vi "Main1.vi"() -> ()   [LabVIEW 2017]
uses:
  <vilib>/Analysis/baseanly.llb/Mean (DBL).vi
  <vilib>/Analysis/NI_AALBase.lvlib
panel:
  out "file path":path=path "M:/Oceanoptics/TDMS test/Spectrometer_test213.tdms"
  out "Image Out":T1(plugin-control)
  out "String":string
  in  "Save Raw Spectrometer Data":bool=TRUE
  out "Spectrometer Data":T2={[750.0, 800.0], "mean"=-22.554463094146342, array[2540 elements], array[2540 elements], "Color Temperatures"=[[-3182.0998200450113], [-4677.963743364752], [-7826.4943596651665]]}
  out "Voltage Average":dbl
  in  "Wait time (ms)":i32=250
  out "Motor Cluster":cluster{"Motor Relative":dbl[]}={"Motor Relative"=[0.0900112499774972, 0.0, 0.0, 0.0]}
  in  "WL2":dbl=800.0 format="%#_13g"
  in  "WL1":dbl=750.0 format="%#_13g"
  in  "Y axis":T3(ring)=enum."Spectrometer intensity"
  in  "Clear data":bool
  in  "Vi Selection":bool[](array[boolean])=[FALSE, TRUE, TRUE, TRUE, FALSE, TRUE]
  in  "base path":path=path "E:/Materials Testing"
  in  "stop":bool
  out "XY Graph":cluster{"magnitude":dbl[], dbl[]}(graph)
  in  "X axis":T4(ring)=enum."Spectrometer Wavelength"
  # "Power Meter"
  # "Spectrometer"
  # "Sensors"
  # "Motor"
  # "Keithley"
  # "Imaging"
  # "Fluke"
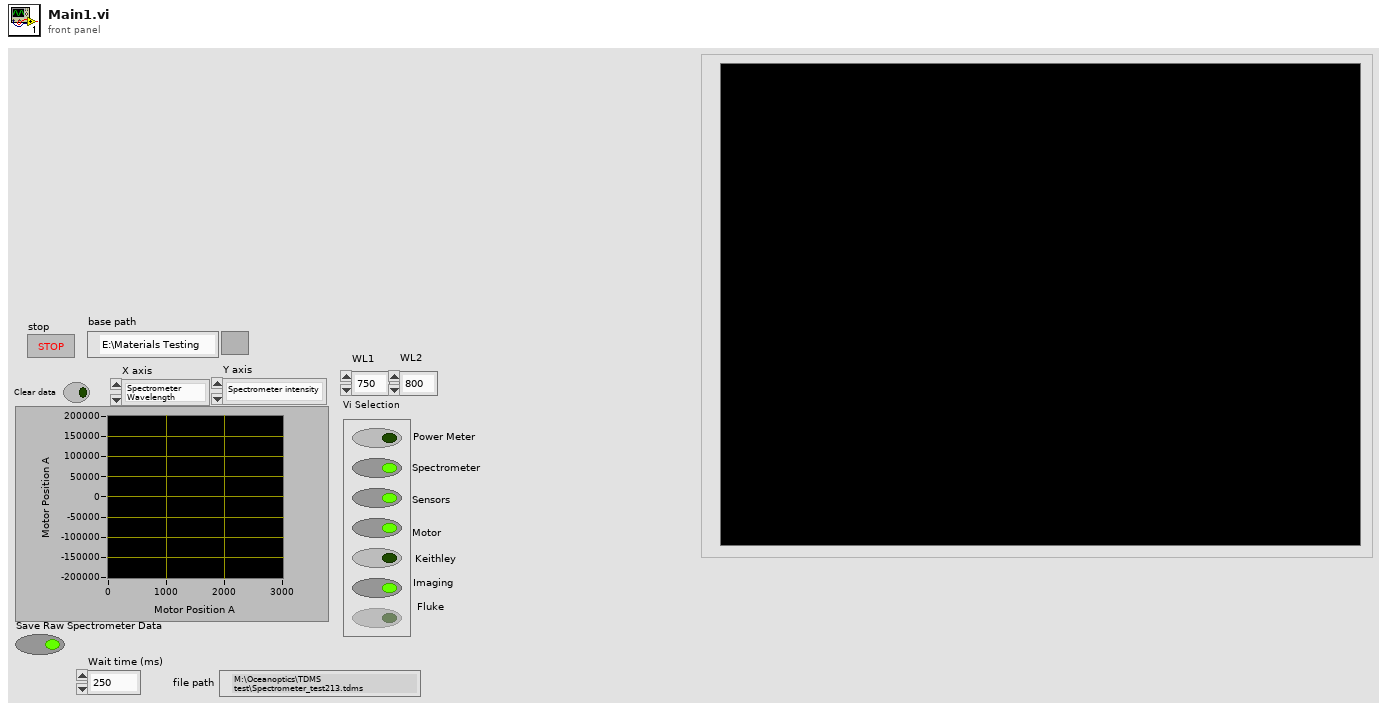
[diagram p1: front panel]
types:
  T1 = typedef "IMAQ Image.ctl" = refnum<image>
  T2 = cluster{dbl[], "mean":dbl, dbl[], dbl[], "Color Temperatures":dbl[][]}
  T3 = enum16{"Motor Position A", "Motor Position B", "Motor Position C", "Motor Position D", "Spectrometer Region Avg.", "Keithley Voltage", "Spectrometer intensity", "Color Temp 2 -3", "Color Temp 1-3", "Color Temp 1-2"}
  T4 = enum16{"Time", "Motor Position A", "Motor Position B", "Motor Position C", "Motor Position D", "Spectrometer Wavelength"}
  T5 = enum16{"PowerMeter", "Spectrometer", "Sensors", "Motor", "Keithley", "Imaging", "Fluke"}
  T6 = enum32{"Invalid", "Standard", "Closed", "Hidden", "Minimized", "Maximized"}
  T7 = cluster{"output cluster 2":cluster{"Value:":dbl[], timestamp[], string[][]}, "output cluster 3":cluster{"Value:":dbl[], timestamp[], string[][]}}
  T8 = cluster{"Temperature Data":cluster{"Bandwidth":i32[], "Bandwidth labels":string[], "Color Temperatures":dbl[][], "Wavelength labels":string[], "seconds since 1Jan1904":timestamp}, "Vis Data":cluster{cluster{"visible wl array":dbl[], dbl[]}, cluster{"Vis or NIR":string, "Multiplexer Response":string, "Wavelength Difference Vis (nm)":dbl, "Vis Integration Time (ms)":u32, "Normalization path":path, "Vis background wave":cluster{dbl[], dbl[]}}}, "NIR Data":cluster{cluster{"NIR wl array":dbl[], dbl[]}, cluster{"Vis or NIR":string, "Multiplexer Response":string, "NIR Integration Time (ms)":u32, "Wavelength Difference NIR (nm) ":dbl, "Normalization path":path, "NIR background wave":cluster{dbl[], dbl[]}}}}
  T9 = cluster{dynamicdata, dynamicdata, dynamicdata, "Dynamic Data Type":dynamicdata}
  T10 = cluster{"Motor Relative":dbl[], "Motor absolute":dbl[], "Motor zero":dbl[], "Time between steps":dbl, "Conversion (steps/mm)":dbl[], "Distance  (mm)":dbl[], "run number":i32, "Number of steps":i32}
  T11 = cluster{"mean":dbl, "seconds since 1Jan1904":timestamp}
  T12 = enum32{"Bad", "Idle", "Run top level", "Running"}
  T13 = cluster{"VI out":refnum<vi>, "error out":errorcluster, refnum<vi>, enum16{"PowerMeter", "Spectrometer", "Sensors", "Motor", "Keithley", "Imaging", "Fluke"}, "Run Power meter":bool}
  T14 = cluster{"Bandwidth":i32[], "Bandwidth labels":string[], "Color Temperatures":dbl[][], "Wavelength labels":string[], "seconds since 1Jan1904":timestamp}
  T15 = cluster{cluster{"visible wl array":dbl[], dbl[]}, cluster{"Vis or NIR":string, "Multiplexer Response":string, "Wavelength Difference Vis (nm)":dbl, "Vis Integration Time (ms)":u32, "Normalization path":path, "Vis background wave":cluster{dbl[], dbl[]}}}
  T16 = cluster{cluster{"NIR wl array":dbl[], dbl[]}, cluster{"Vis or NIR":string, "Multiplexer Response":string, "NIR Integration Time (ms)":u32, "Wavelength Difference NIR (nm) ":dbl, "Normalization path":path, "NIR background wave":cluster{dbl[], dbl[]}}}
  T17 = cluster{"Vis or NIR":string, "Multiplexer Response":string, "NIR Integration Time (ms)":u32, "Wavelength Difference NIR (nm) ":dbl, "Normalization path":path, "NIR background wave":cluster{dbl[], dbl[]}}
  T18 = cluster{"Vis or NIR":string, "Multiplexer Response":string, "Wavelength Difference Vis (nm)":dbl, "Vis Integration Time (ms)":u32, "Normalization path":path, "Vis background wave":cluster{dbl[], dbl[]}}
  T19 = typedef "Image Type" = u32
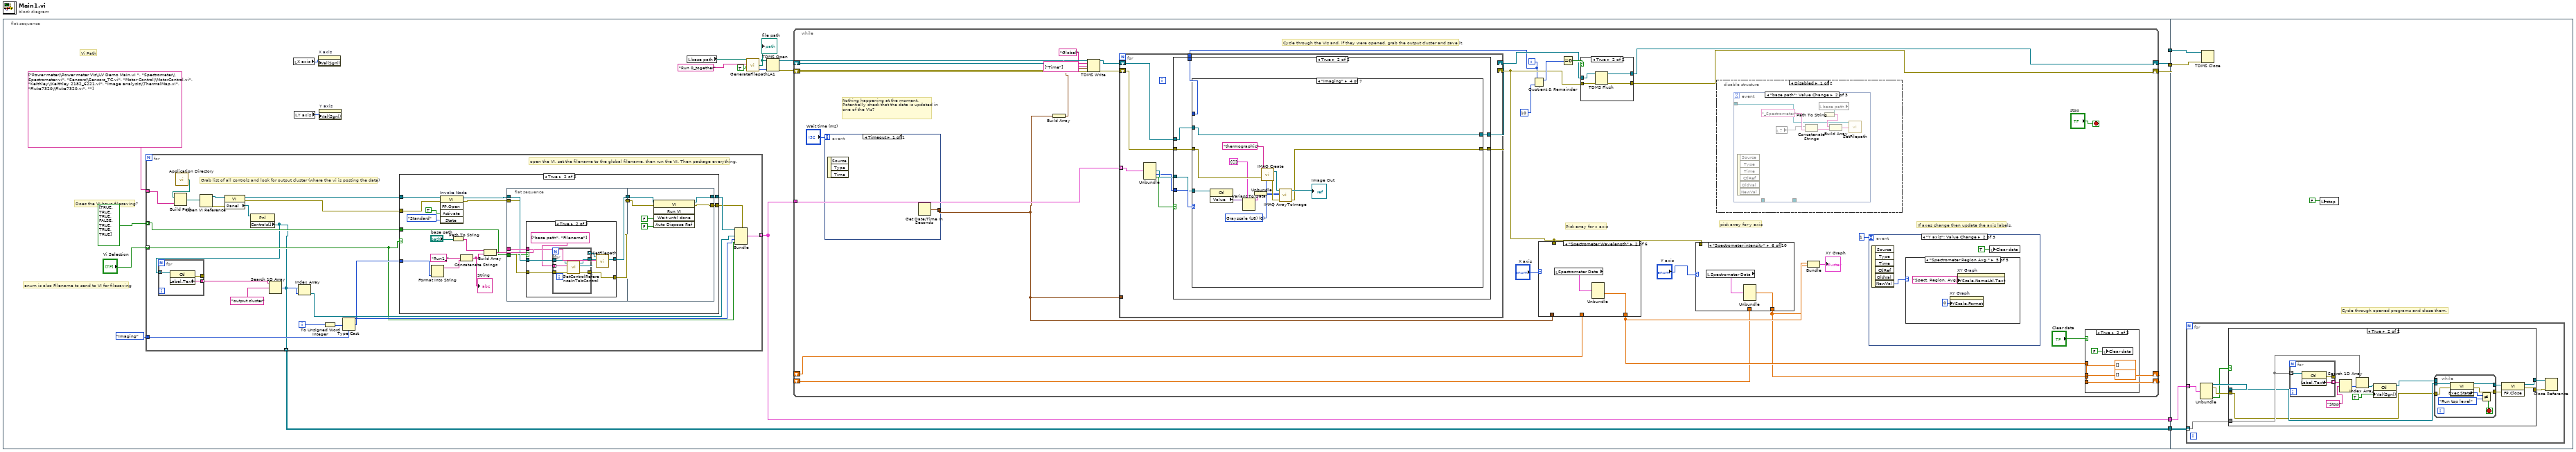
[diagram p0: block diagram]
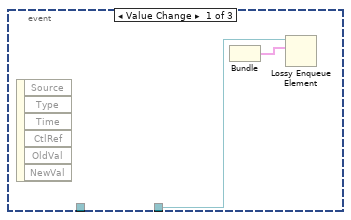
[diagram p5: hidden frame]
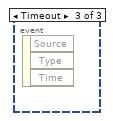
[diagram p6: hidden frame]
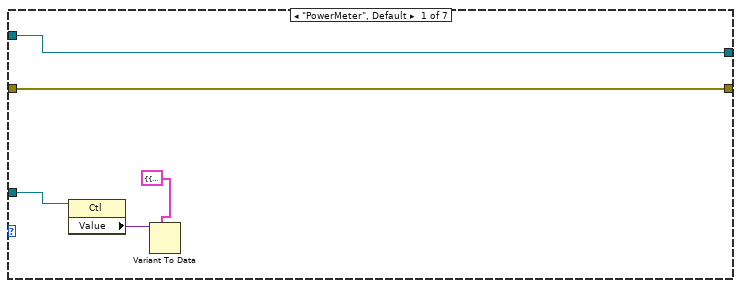
[diagram p9: hidden frame]
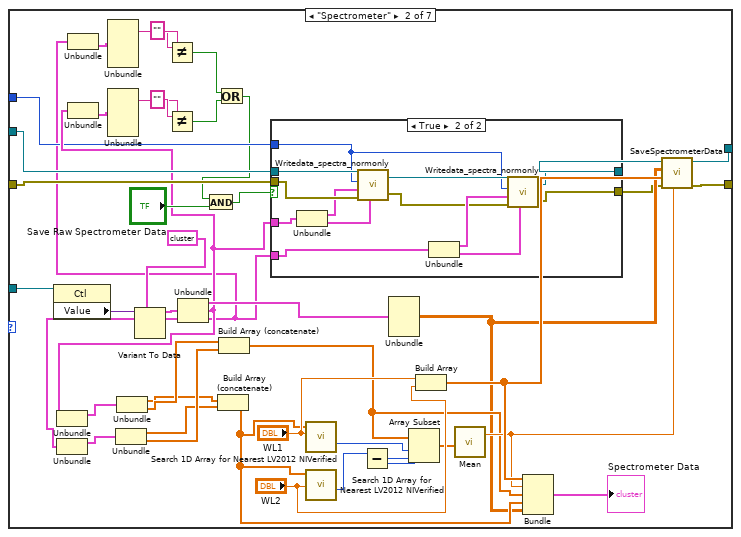
[diagram p10: hidden frame]
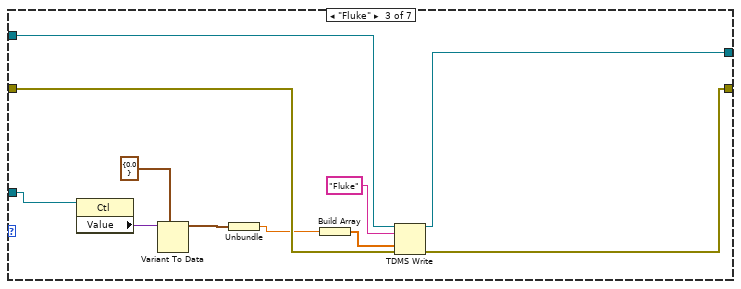
[diagram p12: hidden frame]
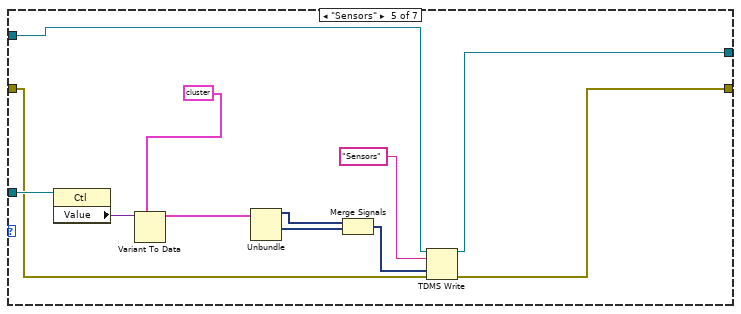
[diagram p13: hidden frame]
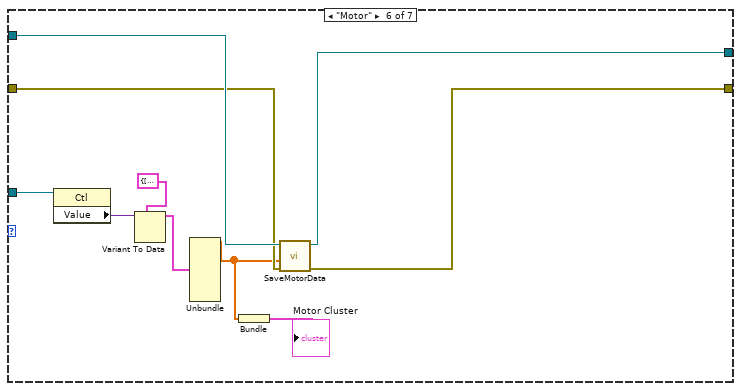
[diagram p14: hidden frame]
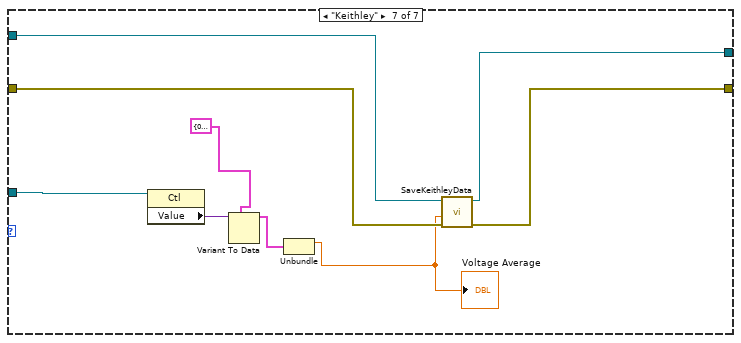
[diagram p15: hidden frame]
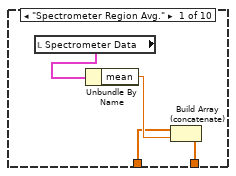
[diagram p17: hidden frame]
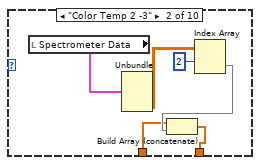
[diagram p18: hidden frame]
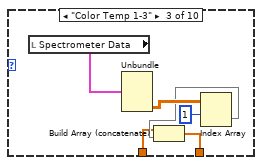
[diagram p19: hidden frame]
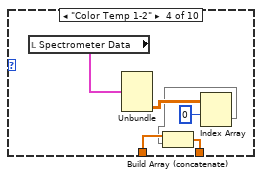
[diagram p20: hidden frame]
diagram:
  n1 = flat-sequence {
    tunnel: [w12] -> w4
    tunnel: [w13] -> w3
    tunnel: [w7] -> w2
    tunnel: [w10] -> w1
    tunnel: w4 -> [w391]
    tunnel: w3 -> [w390]
    tunnel: w2 -> [w389]
    tunnel: w1 -> [w388]
    frame #0 {
      # "Does the VI have filesaving?"
      # "enum is also Filename to send to VI for filesaving"
      # "Vi Path"
      n2 = for {
        tunnel: string[] ["Power meter\\Power meter Vis\\LV Demo Main.vi ", "Spectrometer\\Spectrometer.vi", "Sensors\\Sensors_TC.vi", "Motor Control\\MotorControl.vi", "Keithley\\Keithley 2182_6221.vi", "Image analysis\\ThermalMap.vi", "Fluke7320\\Fluke7320.vi", ""] ("name or relative path") -> [w43] mode=indexing
        tunnel: bool[] [TRUE, TRUE, TRUE, FALSE, TRUE, TRUE, TRUE] ("Vi Selection 2") -> [w25] mode=indexing
        tunnel: T5."Imaging" -> [w42]
        tunnel: [w22] -> w7 mode=indexing
        tunnel: "Vi Selection" -> [w24] mode=indexing
        tunnel: [w23] -> w10 mode=indexing
        i -> [w41]
        # "open the VI, set the filename to the global filename, then run the VI. Then package everything."
        # "Grab list of all controls and look for output cluster (where the vi is posting the data)"
        n3 = call <vilib>:"Application Directory.vi"() -> ("Application Directory"=w36:path)
        n4 = Build Path(base path=w36, name or relative path=w43) -> (appended path=w32:path)
        n5 = Open VI Reference(vi path=w32) -> (vi reference=w34:refnum<vi>, error out=w35:errorcluster)  [unwired: 5 in]
        n6 = property class="VI"(reference=w34, error in=w35) -> (reference out=w39:refnum<vi>, error out=w37:errorcluster, "Panel"=w40:refnum<vi>)
        n7 = property class="Pnl"(reference=w40) -> ("Controls[]"=w23:refnum<vi>[])  [unwired: 1 in, 2 out]
        n8 = for {
          tunnel: w23 -> [w93] mode=indexing
          tunnel: [w92] -> w38 mode=indexing
          tunnel: [w91] -> _
          n9 = property class="Ctl"(reference=w93) -> (error out=w91:errorcluster, "Label.Text"=w92:string)  [unwired: 1 in, 1 out]
        }
        n10 = Search 1D Array(1D array=w38, element="output cluster") -> (index of element=w33:i32)  [unwired: 1 in]
        n11 = Index Array(array=w23, index=w33) -> (element=w27:refnum<vi>)
        n12 = To Unsigned Word Integer(number=w41) -> (unsigned 16bit integer=w28:u16)
        n13 = Type Cast(type=w42, x=w28) -> (*(type *) &x=w26:T5)
        n14 = case shown="True" w24 {
          tunnel: [w45 w58] -> w30
          tunnel: [w44 w57] -> w29
          tunnel: w39 -> [w45 w54]
          tunnel: w37 -> [w44 w53]
          tunnel: w26 -> [_ w50]
          tunnel: w25 -> [_ w49]
          frame False {
          }
          frame True {
            n15 = Format Into String(w50) -> (resulting string=w46:string)  [unwired: 3 in, 1 out]
            n16 = invoke on="Invoke Node" class="VI" method="FP.Open"(reference=w54, error in=w53, "Activate"=TRUE ("Activate?"), "State"=T6."Standard") -> (reference out=w52:refnum<vi>, error out=w51:errorcluster)  [unwired: 1 in, 3 out]
            n17 = Path To String(path="base path") -> (string=w60:string)
            n18 = Concatenate Strings("Run1_" ("string"), w46) -> (w48:string)
            "String" <- w48
            n19 = Build Array(w60, w48) -> (w61:string[])
            n20 = flat-sequence {
              tunnel: w51 -> [w67]
              tunnel: w61 -> [w69]
              tunnel: w52 -> [w68]
              tunnel: [w66] -> w63
              tunnel: [w65] -> w62
              tunnel: w49 -> [w64]
              tunnel: w63 -> [w88]
              tunnel: w62 -> [w86]
              tunnel: [w87] -> w58
              tunnel: [w85] -> w57
              frame #0 {
                n21 = case shown="True" w64 {
                  tunnel: w69 -> [_ w78]
                  tunnel: w68 -> [w71 w76]
                  tunnel: w67 -> [w70 w75]
                  tunnel: [w71 w73] -> w66
                  tunnel: [w70 w72] -> w65
                  frame False {
                  }
                  frame True {
                    n22 = for {
                      tunnel: string[] ["base path", "Filename"] -> [w84] mode=indexing
                      tunnel: w76 -> [w83]
                      tunnel: w75 -> [w82]
                      tunnel: [w81] -> w73
                      tunnel: [w80] -> w72
                      tunnel: [w79] -> w77 mode=indexing
                      n23 = call "GetControlReferenceInTabControl.vi"("error in (no error)"=w82, "Control Name"=w84, "VI in"=w83) -> ("error out"=w80:errorcluster, "Ctl Refnum"=w79:refnum<vi>, "VI out"=w81:refnum<vi>)  [unwired: 6 in]
                    }
                    n24 = call "SetFilepath.vi"("Array 2"=w78, "Array"=w77) -> ()  [unwired: 10 in]
                  }
                }
              }
              frame #1 {
                n25 = invoke class="VI" method="Run VI"(reference=w88, error in=w86, "Wait until done"=FALSE ("Wait Until Done"), "Auto Dispose Ref"=FALSE ("Auto Dispose Reference")) -> (reference out=w87:refnum<vi>, error out=w85:errorcluster)  [unwired: 1 in, 3 out]
              }
            }
          }
        }
        n26 = Bundle("VI out"=w30, "error out"=w29, w27, w26, "Run Power meter"=w24) -> (w22:T13)  [unwired: 1 in]
      }
      n27 = local read "X axis"() -> (w9:T4)
      n28 = local read "Y axis"() -> (w8:T3)
      n29 = property on="X axis" class="Enum (strict)"("Val(Sgnl)"=w9) -> ()  [unwired: 2 in, 2 out]
      n30 = property on="Y axis" class="Enum (strict)"("Val(Sgnl)"=w8) -> ()  [unwired: 2 in, 2 out]
      n31 = local read "base path"() -> (w19:path)
      n32 = call "GenerateFilepathLA1.vi"("Auto Date folder"=TRUE, "Filename"="Run 0_together" ("string"), "base path"=w19) -> ("Numeric"=w20:i32, "file path"=w5:path)  [unwired: 1 in, 1 out]
      "file path" <- w5
      n33 = TDMS Open(10:w20, 11:w5) -> (0:w18:errorcluster, 3:w17:refnum<k34>)  [unwired: 5 in]
      n34 = while {
        shift-right: [w103] -> w13
        shift-left: w17 -> [w112]
        shift-right: [w102] -> w12
        shift-left: w18 -> [w113]
        tunnel: w7 -> [w116]
        shift-right: [w105] -> _
        shift-left: _ -> [w97]
        shift-right: [w106] -> _
        shift-left: _ -> [w95]
        i -> [w94]
        stop <- "stop" stop-if-true
        # "If axes change then update the axis labels."
        # "pick array for y axis"
        # "Pick array for x axis"
        # "Cycle through the VIs and, if they were opened, grab the output cluster and save it."
        # "Nothing happening at the moment. Potentially check that the data is updated in one of the VIs?"
        n35 = event shown="[0] Timeout" {
          selector: _ -> [_]
          dyn-events: _ -> [_]
          timeout: "Wait time (ms)" -> [_]
          tunnel: [w124] -> w100
          event Timeout {
            n36 = event-data() -> ()  [unwired: 1 in, 3 out]
            n37 = Get Date/Time In Seconds() -> (seconds since 1Jan1904=w124:timestamp)
          }
        }
        n38 = Build Array(w100) -> (w111:timestamp[])
        n39 = TDMS Write(0:w112, 5:"Global" ("group name in (Untitled)"), 7:string[] ["Time"] ("channel name(s) in (Untitled)"), 9:w111, 11:w113) -> (4:w108:refnum<k34>, 15:w107:errorcluster)  [unwired: 1 in, 2 out]
        n40 = for {
          tunnel: w116 -> [w149] mode=indexing
          shift-right: [w146] -> w115
          shift-left: w108 -> [w148]
          shift-right: [w145] -> w101
          shift-left: w107 -> [w147]
          tunnel: w100 -> [_]
          tunnel: w94 -> [w141]
          n41 = Unbundle(w149) -> (w144:refnum<vi>, w143:T5, "Run Power meter"=w142:bool)  [unwired: 2 out]
          n42 = case shown="True" w142 {
            tunnel: w143 -> [_ w158]
            tunnel: w144 -> [_ w157]
            tunnel: w148 -> [w151 w156]
            tunnel: w147 -> [w150 w155]
            tunnel: [w151 w154] -> w146
            tunnel: [w150 w153] -> w145
            tunnel: w141 -> [_ w152]
            frame False {
            }
            frame True {
              n43 = case shown="\"Imaging\"" w158 {
                tunnel: w157 -> [w162 w206 w231 w245 w257 w267 w274]
                tunnel: w156 -> [w160 w179 w229 w243 w254 w263 w273]
                tunnel: w155 -> [w159 w178 w228 w237 w253 w261 w272]
                tunnel: [w160 w198 w224 w243 w250 w262 w271] -> w154
                tunnel: [w159 w197 w223 w235 w252 w260 w270] -> w153
                tunnel: w152 -> [_ w171 _ _ _ _ _]
                frame "PowerMeter", Default {
                  n44 = property class="Ctl"(reference=w162) -> ("Value"=w163:variant)  [unwired: 1 in, 2 out]
                  n45 = Variant To Data(type=T7 {"output cluster 2"={"Value:"=[], [], []}, "output cluster 3"={"Value:"=[], [], []}} ("Power meter Cluster 2"), Variant=w163) -> ()  [unwired: 1 in, 2 out]
                }
                frame "Spectrometer" {
                  n46 = property class="Ctl"(reference=w206) -> ("Value"=w205:variant)  [unwired: 1 in, 2 out]
                  n47 = Variant To Data(type=T8 {"Temperature Data"={"Bandwidth"=[10, 10, 10], "Bandwidth labels"=["Bandwidth 1-2", "Bandwidth 2-3", "Bandwidth 1-3"], "Color Temperatures"=[[879.3311636229715], [-21903.619530261916], [-1063.75969736004]], "Wavelength labels"=["Temp1050-1120", "Temp1050-1230", "Temp1120-1230"], "seconds since 1Jan1904"=timestamp(3594756427.269044 s since 1904-01-01)}, "Vis Data"={{"visible wl array"=array[512 elements], array[512 elements]}, {"Vis or NIR"="NIR", "Multiplexer Response"="-1", "Wavelength Difference Vis (nm)"=50.0, "Vis Integration Time (ms)"=100, "Normalization path"=path "E:/Materials Testing/Calibration/2017-11-09/Multiplexter.tdms", "Vis background wave"={array[512 elements], array[512 elements]}}}, "NIR Data"={{"NIR wl array"=array[2028 elements], array[2028 elements]}, {"Vis or NIR"="Visible", "Multiplexer Response"="-1", "NIR Integration Time (ms)"=100, "Wavelength Difference NIR (nm) "=100.0, "Normalization path"=path "E:/Materials Testing/Calibration/2017-11-09/Multiplexter.tdms", "NIR background wave"={array[2028 elements], array[2028 elements]}}}} ("output cluster"), Variant=w205) -> (data=w194:T8)  [unwired: 1 in, 1 out]
                  n48 = Unbundle(w194) -> ("Temperature Data"=w180:T14, "Vis Data"=w172:T15, "NIR Data"=w167:T16)
                  n49 = Unbundle(w172) -> (w186:cluster{"visible wl array":dbl[], dbl[]})  [unwired: 1 out]
                  n50 = Unbundle(w167) -> (w185:cluster{"NIR wl array":dbl[], dbl[]})  [unwired: 1 out]
                  n51 = Unbundle(w167) -> (w169:T17)  [unwired: 1 out]
                  n52 = Unbundle(w172) -> (w174:T18)  [unwired: 1 out]
                  n53 = Unbundle(w169) -> ("Multiplexer Response"=w170:string)  [unwired: 5 out]
                  n54 = Unbundle(w174) -> ("Multiplexer Response"=w173:string)  [unwired: 5 out]
                  n55 = Unbundle(w185) -> ("NIR wl array"=w181:dbl[], w183:dbl[])
                  n56 = Unbundle(w186) -> ("visible wl array"=w182:dbl[], w184:dbl[])
                  n57 = Not Equal?(x="", y=w170) -> (x != y?=w166:bool)
                  n58 = Not Equal?(x="", y=w173) -> (x != y?=w165:bool)
                  n59 = Or(x=w166, y=w165) -> (x .or. y?=w164:bool)
                  n60 = And(x=w164, y="Save Raw Spectrometer Data") -> (x .and. y?=w175:bool)
                  n61 = Build Array (concatenate)(w182, w181) -> (w193:dbl[])
                  n62 = Build Array (concatenate)(w184, w183) -> (w192:dbl[])
                  n63 = case shown="True" w175 {
                    tunnel: [w208 w211] -> w177
                    tunnel: w179 -> [w208 w221]
                    tunnel: [w207 w210] -> w176
                    tunnel: w178 -> [w207 w220]
                    tunnel: w172 -> [_ w219]
                    tunnel: w167 -> [_ w216]
                    tunnel: w171 -> [_ w209]
                    frame False {
                    }
                    frame True {
                      n64 = Unbundle(w219) -> (w218:cluster{"visible wl array":dbl[], dbl[]}, w217:T18)
                      n65 = call "Writedata_spectra_normonly.vi"("tdms file in"=w221, "Aquisition number"=w209, "Norm Visible Intensity"=w218, "tdms error in"=w220, "Params"=w217) -> ("tdms file out"=w213:refnum<k34>, "tdms error out"=w212:errorcluster)
                      n66 = Unbundle(w216) -> (w215:cluster{"NIR wl array":dbl[], dbl[]}, w214:T17)
                      n67 = call "Writedata_spectra_normonly.vi"("tdms file in"=w213, "Aquisition number"=w209, "Norm Visible Intensity"=w215, "tdms error in"=w212, "Params"=w214) -> ("tdms file out"=w211:refnum<k34>, "tdms error out"=w210:errorcluster)
                    }
                  }
                  n68 = call "Search 1D Array for Nearest LV2012 NIVerified.vi"("desired element"="WL1", "1D Array"=w193) -> ("closest index"=w199:i32)  [unwired: 8 in, 1 out]
                  n69 = call "Search 1D Array for Nearest LV2012 NIVerified.vi"("desired element"="WL2", "1D Array"=w193) -> ("closest index"=w200:i32)  [unwired: 8 in, 1 out]
                  n70 = Subtract(x=w200, y=w199) -> (x-y=w201:i32)
                  n71 = Unbundle(w180) -> ("Color Temperatures"=w188:dbl[][])  [unwired: 4 out]
                  n72 = Array Subset(array=w192, index=w199, length=w201) -> (w202:dbl[])
                  n73 = Build Array("WL1", "WL2") -> (w196:dbl[])
                  n74 = call-poly <vilib>:"Mean.vi"("X"=w202) -> ("mean"=w195:dbl)  [unwired: 1 out]
                  n75 = Bundle(w196, "mean"=w195, w192, w193, "Color Temperatures"=w188) -> (→"Spectrometer Data":T2)  [unwired: 1 in]
                  n76 = call "SaveSpectrometerData.vi"("Average"=w195, "error in (no error)"=w176, "Wavelengths"=w196, "Color Temperatures"=w188, "Refnum in"=w177) -> ("error out"=w197:errorcluster, "Refnum out"=w198:refnum<k34>)  [unwired: 5 in]
                }
                frame "Fluke" {
                  n77 = property class="Ctl"(reference=w231) -> ("Value"=w232:variant)  [unwired: 1 in, 2 out]
                  n78 = Variant To Data(type=cluster{dbl} {0.0} ("output cluster"), Variant=w232) -> (data=w227:cluster{dbl})  [unwired: 1 in, 1 out]
                  n79 = Unbundle(w227) -> (w225:dbl)
                  n80 = Build Array(w225) -> (w226:dbl[])
                  n81 = TDMS Write(0:w229, 5:"Fluke", 9:w226, 11:w228) -> (4:w224:refnum<k34>, 15:w223:errorcluster)  [unwired: 2 in, 2 out]
                }
                frame "Imaging" {
                  w240 = T19 0 items=["Grayscale (U8)", "Grayscale (I16)", "Grayscale (SGL)", "Complex (CSG)", "RGB (U32)", "HSL (U32)", "RGB (U64)", "Grayscale (U16)"] ("Image Type")
                  n82 = property class="Ctl"(reference=w245) -> ("Value"=w244:variant)  [unwired: 1 in, 2 out]
                  n83 = Variant To Data(type=cluster{"Image Pixels (U8)":u8[][]} {"Image Pixels (U8)"=[]} ("output cluster"), Variant=w244) -> (data=w242:cluster{"Image Pixels (U8)":u8[][]})  [unwired: 1 in, 1 out]
                  n84 = Unbundle(w242) -> ("Image Pixels (U8)"=w233:u8[][])
                  n85 = call "IMAQ Create"("Image Name"="thermographic", "Image Type"=w240, "error in (no error)"=w237) -> ("New Image"=w241:T1, "error out"=w236:errorcluster)  [unwired: 2 in]
                  n86 = call "IMAQ ArrayToImage"("error in (no error)"=w236, "Image Pixels (U8)"=w233, "Image"=w241) -> ("error out"=w235:errorcluster, "Image Out"=→"Image Out":T1)  [unwired: 7 in]
                }
                frame "Sensors" {
                  n87 = property class="Ctl"(reference=w257) -> ("Value"=w256:variant)  [unwired: 1 in, 2 out]
                  n88 = Variant To Data(type=T9 {[], [], [], "Dynamic Data Type"=[]} ("output cluster"), Variant=w256) -> (data=w255:T9)  [unwired: 1 in, 1 out]
                  n89 = Unbundle(w255) -> (w249:dynamicdata, w248:dynamicdata)  [unwired: 2 out]
                  n90 = Merge Signals(w249, w248) -> (w247:dynamicdata)
                  n91 = TDMS Write(0:w254, 5:"Sensors" ("group name in (Untitled)"), 9:w247, 11:w253) -> (4:w250:refnum<k34>, 15:w252:errorcluster)  [unwired: 2 in, 2 out]
                }
                frame "Motor" {
                  n92 = property class="Ctl"(reference=w267) -> ("Value"=w266:variant)  [unwired: 1 in, 2 out]
                  n93 = Variant To Data(type=T10 {"Motor Relative"=[], "Motor absolute"=[], "Motor zero"=[], "Time between steps"=0.0, "Conversion (steps/mm)"=[], "Distance  (mm)"=[], "run number"=0, "Number of steps"=0} ("output cluster 2"), Variant=w266) -> (data=w265:T10)  [unwired: 1 in, 1 out]
                  n94 = Unbundle(w265) -> ("Motor Relative"=w258:dbl[])  [unwired: 7 out]
                  n95 = Bundle("Motor Relative"=w258) -> (→"Motor Cluster":cluster{"Motor Relative":dbl[]})  [unwired: 1 in]
                  n96 = call "SaveMotorData.vi"("error in (no error)"=w261, "Motor Relative"=w258, "Refnum in"=w263) -> ("error out"=w260:errorcluster, "Refnum out"=w262:refnum<k34>)  [unwired: 7 in]
                }
                frame "Keithley" {
                  n97 = property class="Ctl"(reference=w274) -> ("Value"=w276:variant)  [unwired: 1 in, 2 out]
                  n98 = Variant To Data(type=T11 {"mean"=0.0, "seconds since 1Jan1904"=timestamp(0 s since 1904-01-01)} ("output cluster 2"), Variant=w276) -> (data=w275:T11)  [unwired: 1 in, 1 out]
                  n99 = Unbundle(w275) -> ("mean"=w268:dbl)  [unwired: 1 out]
                  "Voltage Average" <- w268
                  n100 = call "SaveKeithleyData.vi"("error in (no error)"=w272, "Voltage average"=w268, "Refnum in"=w273) -> ("error out"=w270:errorcluster, "Refnum out"=w271:refnum<k34>)  [unwired: 7 in]
                }
              }
            }
          }
        }
        n101 = Quotient & Remainder(x=w94, y=10) -> (x-y*floor(x/y)=w117:i32)  [unwired: 1 out]
        n102 = case shown="\"Spectrometer Wavelength\"" "X axis" {
          tunnel: w100 -> [w337 _ _ _ _ _]
          tunnel: w101 -> [_ _ _ _ _ _]
          tunnel: [w335 w338 w340 w347 w353 w358] -> w98
          tunnel: w97 -> [w334 _ w341 w346 w352 w359]
          frame "Time" {
            n103 = To Double Precision Float(number=w337) -> (double precision float=w336:dbl)
            n104 = Build Array (concatenate)(w334, w336) -> (w335:dbl[])
          }
          frame "Spectrometer Wavelength" {
            n105 = local read "Spectrometer Data"() -> (w339:T2)
            n106 = Unbundle(w339) -> (w338:dbl[])  [unwired: 4 out]
          }
          frame "Motor Position A" {
            n107 = local read "Motor Cluster"() -> (w345:cluster{"Motor Relative":dbl[]})
            n108 = Unbundle By Name(w345) -> ("Motor Relative"=w344:dbl[])
            n109 = Index Array(array=w344, index=0 ("disabled index (col)")) -> (element=w342:dbl)
            n110 = Build Array (concatenate)(w341, w342) -> (w340:dbl[])
          }
          frame "Motor Position B" {
            n111 = local read "Motor Cluster"() -> (w351:cluster{"Motor Relative":dbl[]})
            n112 = Unbundle By Name(w351) -> ("Motor Relative"=w350:dbl[])
            n113 = Index Array(array=w350, index=1 ("disabled index (col)")) -> (element=w348:dbl)
            n114 = Build Array (concatenate)(w346, w348) -> (w347:dbl[])
          }
          frame "Motor Position C" {
            n115 = local read "Motor Cluster"() -> (w357:cluster{"Motor Relative":dbl[]})
            n116 = Unbundle By Name(w357) -> ("Motor Relative"=w356:dbl[])
            n117 = Index Array(array=w356, index=2 ("disabled index (col)")) -> (element=w354:dbl)
            n118 = Build Array (concatenate)(w352, w354) -> (w353:dbl[])
          }
          frame "Motor Position D" {
            n119 = local read "Motor Cluster"() -> (w363:cluster{"Motor Relative":dbl[]})
            n120 = Unbundle By Name(w363) -> ("Motor Relative"=w362:dbl[])
            n121 = Index Array(array=w362, index=3 ("disabled index (col)")) -> (element=w360:dbl)
            n122 = Build Array (concatenate)(w359, w360) -> (w358:dbl[])
          }
        }
        n123 = Equal To 0?(x=w117) -> (x = 0?=w118:bool)
        n124 = case shown="True" w118 {
          tunnel: [w277 w282] -> w103
          tunnel: [w278 w281] -> w102
          tunnel: w101 -> [w278 w280]
          tunnel: w115 -> [w277 w279]
          frame False {
          }
          frame True {
            n125 = TDMS Flush(4:w280, 7:w279) -> (0:w281:errorcluster, 3:w282:refnum<k34>)
          }
        }
        n126 = case shown="\"Spectrometer intensity\"" "Y axis" {
          tunnel: w101 -> [_ _ _ _ _ _ _ _ _ _]
          tunnel: [w284 w289 w295 w299 w305 w308 w310 w316 w322 w328] -> w96
          tunnel: w95 -> [w283 w287 w293 w301 w306 _ w311 w317 w323 w329]
          frame "Spectrometer Region Avg." {
            n127 = local read "Spectrometer Data"() -> (w286:T2)
            n128 = Unbundle By Name(w286) -> ("mean"=w285:dbl)
            n129 = Build Array (concatenate)(w283, w285) -> (w284:dbl[])
          }
          frame "Color Temp 2 -3" {
            n130 = local read "Spectrometer Data"() -> (w292:T2)
            n131 = Unbundle(w292) -> ("Color Temperatures"=w291:dbl[][])  [unwired: 4 out]
            n132 = Index Array(array=w291, index (row)=2) -> (element=w288:dbl[])  [unwired: 1 in]
            n133 = Build Array (concatenate)(w287, w288) -> (w289:dbl[])
          }
          frame "Color Temp 1-3" {
            n134 = local read "Spectrometer Data"() -> (w298:T2)
            n135 = Unbundle(w298) -> ("Color Temperatures"=w297:dbl[][])  [unwired: 4 out]
            n136 = Index Array(array=w297, index (row)=1) -> (element=w294:dbl[])  [unwired: 1 in]
            n137 = Build Array (concatenate)(w293, w294) -> (w295:dbl[])
          }
          frame "Color Temp 1-2" {
            n138 = local read "Spectrometer Data"() -> (w304:T2)
            n139 = Unbundle(w304) -> ("Color Temperatures"=w303:dbl[][])  [unwired: 4 out]
            n140 = Index Array(array=w303, index (row)=0) -> (element=w300:dbl[])  [unwired: 1 in]
            n141 = Build Array (concatenate)(w301, w300) -> (w299:dbl[])
          }
          frame "Keithley Voltage" {
            n142 = local read "Voltage Average"() -> (w307:dbl)
            n143 = Build Array (concatenate)(w306, w307) -> (w305:dbl[])
          }
          frame "Spectrometer intensity" {
            n144 = local read "Spectrometer Data"() -> (w309:T2)
            n145 = Unbundle(w309) -> (w308:dbl[])  [unwired: 4 out]
          }
          frame "Motor Position D" {
            n146 = local read "Motor Cluster"() -> (w313:cluster{"Motor Relative":dbl[]})
            n147 = Unbundle By Name(w313) -> ("Motor Relative"=w314:dbl[])
            n148 = Index Array(array=w314, index=3 ("disabled index (col)")) -> (element=w312:dbl)
            n149 = Build Array (concatenate)(w311, w312) -> (w310:dbl[])
          }
          frame "Motor Position C" {
            n150 = local read "Motor Cluster"() -> (w319:cluster{"Motor Relative":dbl[]})
            n151 = Unbundle By Name(w319) -> ("Motor Relative"=w320:dbl[])
            n152 = Index Array(array=w320, index=2 ("disabled index (col)")) -> (element=w318:dbl)
            n153 = Build Array (concatenate)(w317, w318) -> (w316:dbl[])
          }
          frame "Motor Position B" {
            n154 = local read "Motor Cluster"() -> (w325:cluster{"Motor Relative":dbl[]})
            n155 = Unbundle By Name(w325) -> ("Motor Relative"=w326:dbl[])
            n156 = Index Array(array=w326, index=1 ("disabled index (col)")) -> (element=w324:dbl)
            n157 = Build Array (concatenate)(w323, w324) -> (w322:dbl[])
          }
          frame "Motor Position A" {
            n158 = local read "Motor Cluster"() -> (w331:cluster{"Motor Relative":dbl[]})
            n159 = Unbundle By Name(w331) -> ("Motor Relative"=w332:dbl[])
            n160 = Index Array(array=w332, index=0 ("disabled index (col)")) -> (element=w330:dbl)
            n161 = Build Array (concatenate)(w329, w330) -> (w328:dbl[])
          }
        }
        n162 = disable-structure shown="Disabled" {
          frame Disabled {
            n163 = event shown="[1] \"base path\": Value Change" {
              selector: _ -> [_ _ _]
              dyn-events: _ -> [_ _ _]
              timeout: _ -> [_ _ _]
              tunnel: _ -> [_ _ _]
              tunnel: _ -> [_ w134 _]
              tunnel: _ -> [w132 _ _]
              event Value Change {
                n164 = event-data() -> ("NewVal"=w133:variant)  [unwired: 1 in, 5 out]
                n165 = Bundle() -> (w131:cluster{void, void}, w130)  [unwired: 2 in]
                n166 = Lossy Enqueue Element(queue=w132, element=w131) -> ()  [unwired: 1 in, 4 out]
              }
              event "base path": Value Change {
                n167 = event-data() -> ()  [unwired: 1 in, 6 out]
                n168 = local read item#-1() -> (w137)
                n169 = Concatenate Strings(w137, "_Spectrometer" ("string")) -> (w138:string)
                n170 = local read "base path"() -> (w136:path)
                n171 = Path To String(path=w136) -> (string=w139:string)
                n172 = Build Array(w139, w138) -> (w135:string[])
                n173 = call "SetFilepath.vi"("Array 2"=w135, "Array"=w134) -> ()  [unwired: 10 in]
              }
              event Timeout {
                n174 = event-data() -> ()  [unwired: 1 in, 3 out]
              }
            }
          }
          frame Enabled {
          }
        }
        n175 = Bundle(w98, w96) -> (→"XY Graph":cluster{dbl[], dbl[]})  [unwired: 1 in]
        n176 = event shown="[1] \"Y axis\": Value Change" {
          selector: _ -> [_ _ _]
          dyn-events: _ -> [_ _ _]
          timeout: 1 -> [_ _ _]
          event "X axis": Value Change {
            n177 = event-data() -> ("NewVal"=w365:T4)  [unwired: 1 in, 5 out]
            n178 = case shown="\"Time\"" w365 {
              frame "Time" {
                n179 = property on="XY Graph" class="XYGraph (strict)"("XScale.Format"=u8 7 ("Y Scale.Display Format:Format")) -> ()  [unwired: 2 in, 2 out]
                n180 = property on="XY Graph" class="XYGraph (strict)"("XScale.NameLbl.Text"="Time" ("X Scale.Name Label.Text")) -> ()  [unwired: 2 in, 2 out]
              }
              frame "Motor Position A", Default {
                n181 = property on="XY Graph" class="XYGraph (strict)"("XScale.Format"=u8 0 ("Y Scale.Display Format:Format")) -> ()  [unwired: 2 in, 2 out]
                n182 = property on="XY Graph" class="XYGraph (strict)"("XScale.NameLbl.Text"="Motor Position A" ("X Scale.Name Label.Text")) -> ()  [unwired: 2 in, 2 out]
              }
              frame "Motor Position B" {
                n183 = property on="XY Graph" class="XYGraph (strict)"("XScale.Format"=u8 0 ("Y Scale.Display Format:Format")) -> ()  [unwired: 2 in, 2 out]
                n184 = property on="XY Graph" class="XYGraph (strict)"("XScale.NameLbl.Text"="Motor Position B" ("X Scale.Name Label.Text")) -> ()  [unwired: 2 in, 2 out]
              }
              frame "Motor Position C" {
                n185 = property on="XY Graph" class="XYGraph (strict)"("XScale.Format"=u8 0 ("Y Scale.Display Format:Format")) -> ()  [unwired: 2 in, 2 out]
                n186 = property on="XY Graph" class="XYGraph (strict)"("XScale.NameLbl.Text"="Motor Position C" ("X Scale.Name Label.Text")) -> ()  [unwired: 2 in, 2 out]
              }
              frame "Motor Position D" {
                n187 = property on="XY Graph" class="XYGraph (strict)"("XScale.Format"=u8 0 ("Y Scale.Display Format:Format")) -> ()  [unwired: 2 in, 2 out]
                n188 = property on="XY Graph" class="XYGraph (strict)"("XScale.NameLbl.Text"="Motor Position D" ("X Scale.Name Label.Text")) -> ()  [unwired: 2 in, 2 out]
              }
            }
            n189 = local write "Clear data"(TRUE ("Clear data")) -> ()
          }
          event "Y axis": Value Change {
            n190 = event-data() -> ("NewVal"=w377:T3)  [unwired: 1 in, 5 out]
            n191 = case shown="\"Spectrometer Region Avg.\"" w377 {
              frame "Motor Position A", Default {
                n192 = property on="XY Graph" class="XYGraph (strict)"("YScale.Format"=u8 0 ("Y Scale.Display Format:Format")) -> ()  [unwired: 2 in, 2 out]
                n193 = property on="XY Graph" class="XYGraph (strict)"("YScale.NameLbl.Text"="Motor Position A" ("X Scale.Name Label.Text")) -> ()  [unwired: 2 in, 2 out]
              }
              frame "Motor Position B" {
                n194 = property on="XY Graph" class="XYGraph (strict)"("YScale.Format"=u8 0 ("Y Scale.Display Format:Format")) -> ()  [unwired: 2 in, 2 out]
                n195 = property on="XY Graph" class="XYGraph (strict)"("YScale.NameLbl.Text"="Motor Position B" ("X Scale.Name Label.Text")) -> ()  [unwired: 2 in, 2 out]
              }
              frame "Motor Position C" {
                n196 = property on="XY Graph" class="XYGraph (strict)"("YScale.Format"=u8 0 ("Y Scale.Display Format:Format")) -> ()  [unwired: 2 in, 2 out]
                n197 = property on="XY Graph" class="XYGraph (strict)"("YScale.NameLbl.Text"="Motor Position C" ("X Scale.Name Label.Text")) -> ()  [unwired: 2 in, 2 out]
              }
              frame "Motor Position D" {
                n198 = property on="XY Graph" class="XYGraph (strict)"("YScale.Format"=u8 0 ("Y Scale.Display Format:Format")) -> ()  [unwired: 2 in, 2 out]
                n199 = property on="XY Graph" class="XYGraph (strict)"("YScale.NameLbl.Text"="Motor Position D" ("X Scale.Name Label.Text")) -> ()  [unwired: 2 in, 2 out]
              }
              frame "Spectrometer Region Avg." {
                n200 = property on="XY Graph" class="XYGraph (strict)"("YScale.Format"=u8 0 ("Y Scale.Display Format:Format")) -> ()  [unwired: 2 in, 2 out]
                n201 = property on="XY Graph" class="XYGraph (strict)"("YScale.NameLbl.Text"="Spect. Region. Avg." ("X Scale.Name Label.Text")) -> ()  [unwired: 2 in, 2 out]
              }
            }
            n202 = local write "Clear data"(TRUE ("Clear data")) -> ()
          }
          event Timeout {
            n203 = event-data() -> ()  [unwired: 1 in, 3 out]
          }
        }
        n204 = case shown="True" "Clear data" {
          tunnel: w98 -> [w125 _]
          tunnel: w96 -> [w126 _]
          tunnel: [w126 dbl[] []] -> w106
          tunnel: [w125 dbl[] []] -> w105
          frame False {
          }
          frame True {
            n205 = local write "Clear data"(FALSE ("Clear data")) -> ()
          }
        }
      }
    }
    frame #1 {
      # "Cycle through opened programs and close them."
      n206 = for {
        tunnel: w389 -> [w398] mode=indexing
        tunnel: w388 -> [w393] mode=indexing
        n207 = Unbundle(w398) -> ("VI out"=w397:refnum<vi>, "error out"=w396:errorcluster, "Run Power meter"=w394:bool)  [unwired: 2 out]
        n208 = case shown="True" w394 {
          tunnel: [w401 w413] -> w399
          tunnel: w397 -> [w401 w404]
          tunnel: w396 -> [w400 w403]
          tunnel: [w400 w412] -> w395
          tunnel: w393 -> [_ w406]
          frame False {
          }
          frame True {
            n209 = for {
              tunnel: w406 -> [w417] mode=indexing
              tunnel: [w416] -> w409 mode=indexing
              tunnel: [w415] -> _
              n210 = property class="Ctl"(reference=w417) -> (error out=w415:errorcluster, "Label.Text"=w416:string)  [unwired: 1 in, 1 out]
            }
            n211 = Search 1D Array(1D array=w409, element="Stop") -> (index of element=w408:i32)  [unwired: 1 in]
            n212 = Index Array(array=w406, index=w408) -> (element=w410:refnum<vi>)
            n213 = property class="Ctl"(reference=w410, "Val(Sgnl)"=TRUE) -> (reference out=w402:refnum<vi>)  [unwired: 1 in, 1 out]
            n214 = while {
              tunnel: w404 -> [w425]
              tunnel: [w424] -> w414
              tunnel: w403 -> [w420]
              tunnel: [w419] -> w411
              tunnel: [w418] -> _
              tunnel: w402 -> [w418]
              stop <- w423 stop-if-true
              n215 = property class="VI"(reference=w425, error in=w420) -> (reference out=w424:refnum<vi>, error out=w419:errorcluster, "Exec.State"=w422:T12)
              n216 = Not Equal?(x=w422, y=T12."Run top level" ("Execution:State 2")) -> (x != y?=w423:bool)
            }
            n217 = invoke class="VI" method="FP.Close"(reference=w414, error in=w411) -> (reference out=w413:refnum<vi>, error out=w412:errorcluster)  [unwired: 1 in, 1 out]
          }
        }
        n218 = Close Reference(reference=w399, error in (no error)=w395) -> ()  [unwired: 1 out]
      }
      n219 = TDMS Close(8:w391, 11:w390) -> ()  [unwired: 2 out]
      n220 = local write "stop"(FALSE ("stop")) -> ()
    }
  }
